vi "음료자판기.vi"() -> ()   [LabVIEW 2014]
panel:
  in  "음료선택":u8(knob) max=2 step=1 scale=0.0..2.0
  in  "정지":bool
  in  "구매":bool
  in  "음료수량초기값":cluster{"콜라":u8, "사이다":u8, "생수":u8}
  out "생수":u8
  out "사이다":u8
  out "콜라":u8
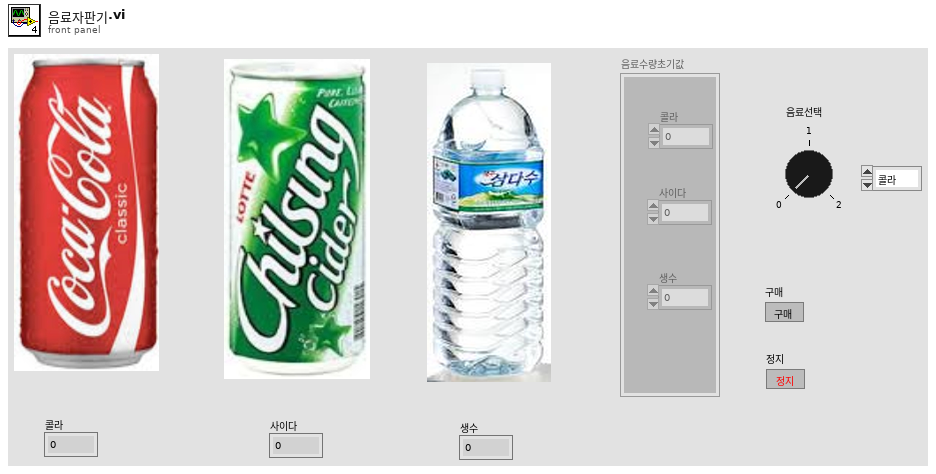
[diagram p1: front panel]
types:
  T1 = typedef "음료.ctl" = enum16{"Idle", "초기화", "정지", "음료확인", "구매"}
  T2 = enum8{"Enabled", "Disabled", "Disabled and Grayed Out"}
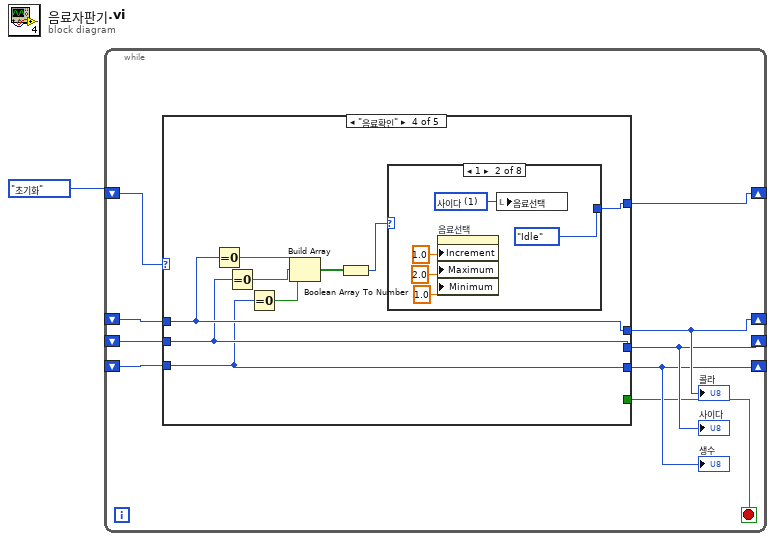
[diagram p0: block diagram]
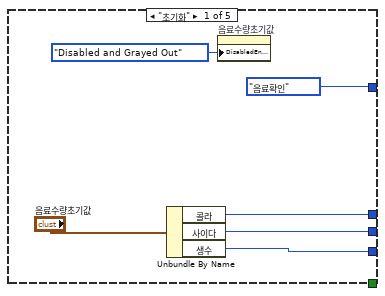
[diagram p2: hidden frame]
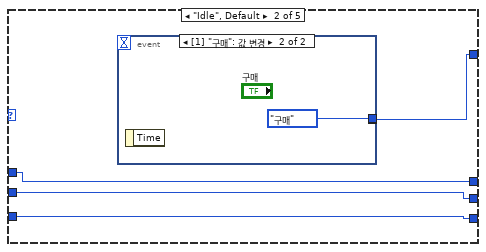
[diagram p3: hidden frame]
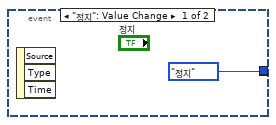
[diagram p4: hidden frame]
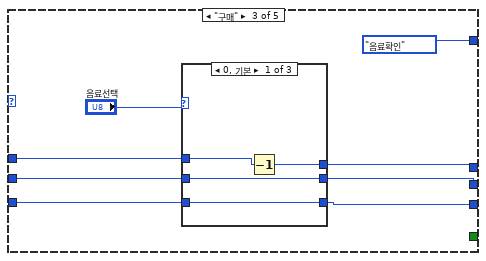
[diagram p5: hidden frame]
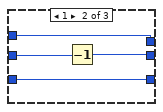
[diagram p6: hidden frame]
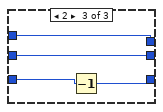
[diagram p7: hidden frame]
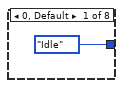
[diagram p8: hidden frame]
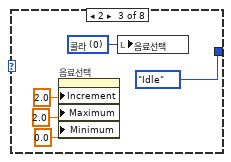
[diagram p9: hidden frame]
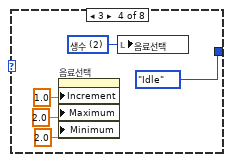
[diagram p10: hidden frame]
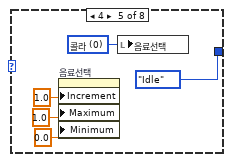
[diagram p11: hidden frame]
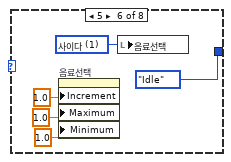
[diagram p12: hidden frame]
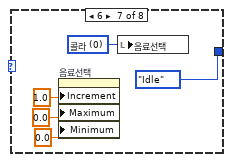
[diagram p13: hidden frame]
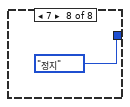
[diagram p14: hidden frame]
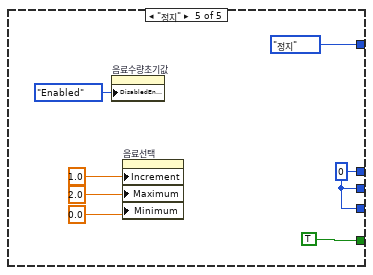
[diagram p15: hidden frame]
diagram:
  n1 = while {
    shift-right: [w10] -> _
    shift-left: 음료."초기화" ("열거형") -> [w2]
    shift-right: [w9] -> _
    shift-left: _ -> [w6]
    shift-right: [w8] -> _
    shift-left: _ -> [w5]
    shift-right: [w7] -> _
    shift-left: _ -> [w4]
    stop <- w3 stop-if-true
    n2 = case shown="\"음료확인\"" w2 {
      tunnel: [음료."음료확인" ("열거형") w20 음료."음료확인" ("열거형") w44 음료."정지" ("열거형")] -> w10
      tunnel: [w14 w19 w27 w51 w84] -> w9
      tunnel: [w13 w18 w24 w50 w84] -> w8
      tunnel: [w12 w17 w23 w43 w84] -> w7
      tunnel: w6 -> [_ w19 w28 w51 _]
      tunnel: w5 -> [_ w18 w26 w50 _]
      tunnel: w4 -> [_ w17 w25 w43 _]
      tunnel: [_ _ _ _ TRUE] -> w3
      frame "초기화" {
        n3 = Unbundle By Name("음료수량초기값") -> ("콜라"=w14:u8, "사이다"=w13:u8, "생수"=w12:u8)
        n4 = property on="음료수량초기값" class="Clust (엄격한)"("DisabledEnum"=T2."Disabled and Grayed Out" ("비활성화")) -> ()  [unwired: 2 in, 2 out]
      }
      frame "Idle", Default {
        n5 = event shown="[1] \"구매\": 값 변경" {
          selector: _ -> [_ _]
          dyn-events: _ -> [_ _]
          timeout: _ -> [_ _]
          tunnel: [음료."정지" ("열거형") _] -> w20
          tunnel: [_ 음료."구매" ("열거형")] -> _
          event "정지": Value Change {
            n6 = event-data() -> ()  [unwired: 1 in, 3 out]
          }
          event "구매": Value Change {
            n7 = event-data() -> ()  [unwired: 1 in, 1 out]
          }
        }
      }
      frame "구매" {
        n8 = case shown="0, 기본" "음료선택" {
          tunnel: w28 -> [w34 w38 w42]
          tunnel: [w33 w38 w42] -> w27
          tunnel: w26 -> [w32 w37 w41]
          tunnel: [w32 w36 w41] -> w24
          tunnel: w25 -> [w31 w35 w40]
          tunnel: [w31 w35 w39] -> w23
          frame 0, Default {
            n9 = Decrement(x=w34) -> (x-1=w33:u8)
          }
          frame 1 {
            n10 = Decrement(x=w37) -> (x-1=w36:u8)
          }
          frame 2 {
            n11 = Decrement(x=w40) -> (x-1=w39:u8)
          }
        }
      }
      frame "음료확인" {
        n12 = Equal To 0?(x=w51) -> (x = 0?=w49:bool)
        n13 = Equal To 0?(x=w50) -> (x = 0?=w48:bool)
        n14 = Equal To 0?(x=w43) -> (x = 0?=w47:bool)
        n15 = Build Array(w49, w48, w47) -> (w46:bool[])
        n16 = Boolean Array To Number(Boolean array=w46) -> (number=w45:u32)
        n17 = case shown="1" w45 {
          tunnel: [음료."Idle" ("열거형") 음료."Idle" ("열거형") 음료."Idle" ("열거형") 음료."Idle" ("열거형") 음료."Idle" ("열거형") 음료."Idle" ("열거형") 음료."Idle" ("열거형") 음료."정지" ("열거형")] -> w44
          frame 0, Default {
          }
          frame 1 {
            w54 = u8 1 items=["콜라", "사이다", "생수"] ("음료선택")
            n18 = property on="음료선택" class="Knob (엄격한)"("Increment"=1.0 ("데이터 입력 제한:증가"), "Maximum"=2.0 ("데이터 입력 제한:최대"), "Minimum"=1.0 ("데이터 입력 제한:최소")) -> ()  [unwired: 2 in, 2 out]
            n19 = local write "음료선택"(w54) -> ()
          }
          frame 2 {
            w59 = u8 0 items=["콜라", "사이다", "생수"] ("음료선택")
            n20 = property on="음료선택" class="Knob (엄격한)"("Increment"=2.0 ("데이터 입력 제한:증가"), "Maximum"=2.0 ("데이터 입력 제한:최대"), "Minimum"=0.0 ("데이터 입력 제한:최소")) -> ()  [unwired: 2 in, 2 out]
            n21 = local write "음료선택"(w59) -> ()
          }
          frame 3 {
            w64 = u8 2 items=["콜라", "사이다", "생수"] ("음료선택")
            n22 = property on="음료선택" class="Knob (엄격한)"("Increment"=1.0 ("데이터 입력 제한:증가"), "Maximum"=2.0 ("데이터 입력 제한:최대"), "Minimum"=2.0 ("데이터 입력 제한:최소")) -> ()  [unwired: 2 in, 2 out]
            n23 = local write "음료선택"(w64) -> ()
          }
          frame 4 {
            w69 = u8 0 items=["콜라", "사이다", "생수"] ("음료선택")
            n24 = property on="음료선택" class="Knob (엄격한)"("Increment"=1.0 ("데이터 입력 제한:증가"), "Maximum"=1.0 ("데이터 입력 제한:최대"), "Minimum"=0.0 ("데이터 입력 제한:최소")) -> ()  [unwired: 2 in, 2 out]
            n25 = local write "음료선택"(w69) -> ()
          }
          frame 5 {
            w74 = u8 1 items=["콜라", "사이다", "생수"] ("음료선택")
            n26 = property on="음료선택" class="Knob (엄격한)"("Increment"=1.0 ("데이터 입력 제한:증가"), "Maximum"=1.0 ("데이터 입력 제한:최대"), "Minimum"=1.0 ("데이터 입력 제한:최소")) -> ()  [unwired: 2 in, 2 out]
            n27 = local write "음료선택"(w74) -> ()
          }
          frame 6 {
            w79 = u8 0 items=["콜라", "사이다", "생수"] ("음료선택")
            n28 = property on="음료선택" class="Knob (엄격한)"("Increment"=1.0 ("데이터 입력 제한:증가"), "Maximum"=0.0 ("데이터 입력 제한:최대"), "Minimum"=0.0 ("데이터 입력 제한:최소")) -> ()  [unwired: 2 in, 2 out]
            n29 = local write "음료선택"(w79) -> ()
          }
          frame 7 {
          }
        }
      }
      frame "정지" {
        w84 = u8 0 ("콜라")
        n30 = property on="음료수량초기값" class="Clust (엄격한)"("DisabledEnum"=T2."Enabled" ("비활성화")) -> ()  [unwired: 2 in, 2 out]
        n31 = property on="음료선택" class="Knob (엄격한)"("Increment"=1.0 ("데이터 입력 제한:증가"), "Maximum"=2.0 ("데이터 입력 제한:최대"), "Minimum"=0.0 ("데이터 입력 제한:최소")) -> ()  [unwired: 2 in, 2 out]
      }
    }
    "콜라" <- w9
    "사이다" <- w8
    "생수" <- w7
  }
